vi "Digital outputs control panel.vi"() -> ()   [LabVIEW 2009]
doc: "A simple VI that lets you manually set digital outputs on a common output device."
uses:
  <vilib>/DAQmx/create/channels.llb/DAQmx Create Channel (DO-Digital Output).vi
  <vilib>/DAQmx/read.llb/DAQmx Read (Digital 2D Bool NChan 1Samp NLine).vi
  <vilib>/DAQmx/create/channels.llb/DAQmx Create Channel (DI-Digital Input).vi
  <vilib>/DAQmx/write.llb/DAQmx Write (Digital 2D Bool NChan 1Samp NLine).vi
panel:
  in  "stop":bool
  in  "data":bool[][](array[boolean])=[[TRUE, TRUE, TRUE, TRUE, TRUE, TRUE, TRUE, TRUE]] caption="0        1       2        3       4        5       6        7"
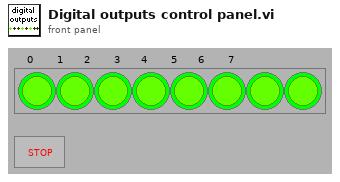
[diagram p1: front panel]
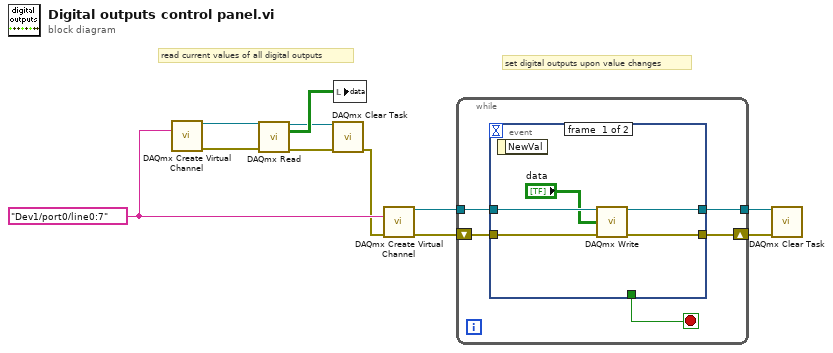
[diagram p0: block diagram]
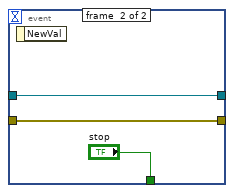
[diagram p2: hidden frame]
diagram:
  w9 = tag "Dev1/port0/line0:7" ("task in")
  # "set digital outputs upon value changes"
  # "read current values of all digital outputs"
  n1 = call-poly <vilib>:"DAQmx Create Virtual Channel.vi"("lines"=w9) -> ("task out"=w8:refnum<k21>, "error out"=w6:errorcluster)  [unwired: 5 in, 8 out]
  n2 = call-poly <vilib>:"DAQmx Read.vi"("task/channels in"=w8, "error in"=w6) -> ("task out"=w5:refnum<k21>, "data"=w7:bool[][], "error out"=w4:errorcluster)  [unwired: 1 in, 10 out]
  n3 = call <vilib>:"DAQmx Clear Task.vi"("task in"=w5, "error in"=w4) -> ("error out"=w1:errorcluster)  [unwired: 13 out]
  n4 = local write "data"(w7) -> ()
  n5 = call-poly <vilib>:"DAQmx Create Virtual Channel.vi"("lines"=w9, "error in"=w1) -> ("task out"=w11:refnum<k21>, "error out"=w10:errorcluster)  [unwired: 4 in, 8 out]
  n6 = while {
    tunnel: w11 -> [w16]
    shift-right: [w14] -> w2
    shift-left: w10 -> [w15]
    tunnel: [w12] -> w3
    stop <- w13 stop-if-true
    n7 = event shown="[1] \"stop\": Value Change" {
      selector: _ -> [_ _]
      dyn-events: _ -> [_ _]
      timeout: _ -> [_ _]
      tunnel: w16 -> [w21 w22]
      tunnel: w15 -> [w20 w23]
      tunnel: [w18 w23] -> w14
      tunnel: [_ "stop"] -> w13
      tunnel: [w17 w22] -> w12
      event #0 {
        n8 = event-data() -> ()  [unwired: 2 out]
        n9 = call-poly <vilib>:"DAQmx Write.vi"("task/channels in"=w21, "data"="data", "error in"=w20) -> ("task out"=w17:refnum<k21>, "error out"=w18:errorcluster)  [unwired: 1 in, 10 out]
      }
      event #1 {
        n10 = event-data() -> ()  [unwired: 2 out]
      }
    }
  }
  n11 = call <vilib>:"DAQmx Clear Task.vi"("task in"=w3, "error in"=w2) -> ()  [unwired: 14 out]
